vi "Asylum_Driver_PostObjectTerminate.vi"(4 "Abort Notifier":refnum<notifier>, 8 "error in (no error)":errorcluster, 9 "Offsets":cluster{"X":dbl, "Y":dbl}, 10 "Pattern Data":T2, 11 "Application In":refnum<k7>) -> (0 "error out":errorcluster, 3 "Application Out":refnum<k7>)   [LabVIEW 2019]
uses:
  <userlib>/LevyLab/Relay Box/Typedefs/Resistor--enum.ctl
  0c3285b1-0af0-47c5-b844-26b55d9538bb.vi
  0c3285b1-0af0-47c5-b844-26b55d9538bb.vi/44aabc3a-2af3-469a-b827-e6af1571d854.vi
  <vilib>/Utility/Debug Log/Display.vi
  <userlib>/LevyLab/Relay Box/Relay-Box.lvclass
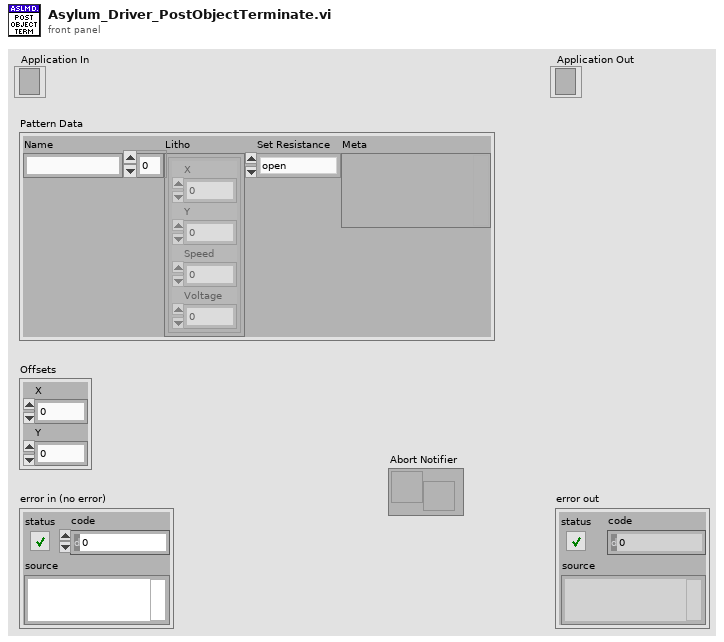
[diagram p1: front panel]
types:
  T1 = typedef "Relay-Box.lvclass/Resistor--enum.ctl" = enum16{"open", "discharge tip", "0 ohms", "100k ohm", "10M ohm", "1G ohm"}
  T2 = cluster{"Name":string, "Litho":cluster{"X":dbl, "Y":dbl, "Speed":dbl, "Voltage":dbl}[], "Set Resistance":T1, "Meta":variant}
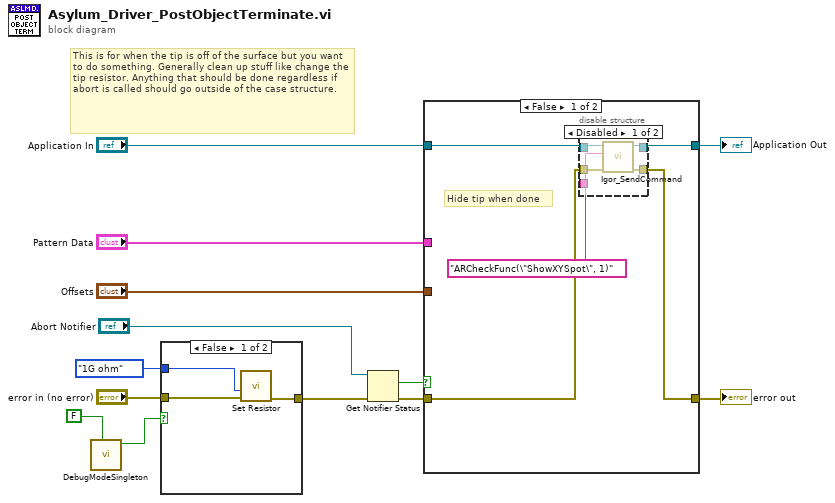
[diagram p0: block diagram]
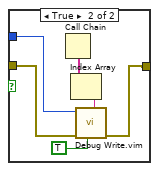
[diagram p2: hidden frame]
diagram:
  # "This is for when the tip is off of the surface but you want to do something. Generally clean up stuff like change the tip resistor. Anything that should be done regardless if abort is called should go outside of the case structure."
  n1 = call <userlib>:"DebugModeSingleton.vi"("Write?"=FALSE) -> ("Debug Mode?"=w2:bool)  [unwired: 10 in]
  n2 = case shown="False" w2 {
    tunnel: "error in (no error)" -> [w16 w17]
    tunnel: [w15 w18] -> w9
    tunnel: Resistor--enum."1G ohm" ("Set Resistance") -> [w14 w19]
    frame False {
      n3 = call <userlib>:"Set Resistor.vi"("error in"=w16, "Set Resistance"=w14) -> ("error out"=w15:errorcluster)  [unwired: 9 in]
    }
    frame True {
      n4 = Call Chain() -> (call chain=w22:string[])
      n5 = Index Array(array=w22) -> (element=w21:string)  [unwired: 1 in]
      n6 = call "Debug Write.vim"("include timestamp? (F)"=TRUE, "prefix (\"\")"=w21, "error in (no error)"=w17, "value"=w19) -> ("error out"=w18:errorcluster)  [unwired: 7 in]
    }
  }
  n7 = Get Notifier Status(notifier="Abort Notifier", error in (no error)=w9) -> (current notification=w6:bool, error out=w8:errorcluster)  [unwired: 3 out]
  n8 = case shown="False" w6 {
    tunnel: "Application In" -> [w27 w36]
    tunnel: [w26 w36] -> w11
    tunnel: [w24 w35] -> w10
    tunnel: w8 -> [w25 w35]
    tunnel: "Pattern Data" -> [_ _]
    tunnel: "Offsets" -> [_ _]
    frame False {
      # "Hide tip when done"
      n9 = disable-structure shown="Disabled" {
        disable-tunnel: w27 -> [w32 w34]
        disable-tunnel: [w31 w34] -> w26
        disable-tunnel: w25 -> [w30 w33]
        disable-tunnel: [w29 w33] -> w24
        disable-tunnel: "ARCheckFunc(\"ShowXYSpot\", 1)" ("parameterName") -> [w28 _]
        frame Disabled {
          n10 = call <userlib>:"Igor_SendCommand.vi"("error in (no error)"=w30, "command"=w28, "Application In"=w32) -> ("error out"=w29:errorcluster, "Application Out"=w31:refnum<k7>)  [unwired: 5 in, 2 out]
        }
        frame Enabled {
        }
      }
    }
    frame True {
      # "Abort has been called. Do nothing new here"
    }
  }
  "error out" <- w10
  "Application Out" <- w11
